vi "Save Config.vi"(8 "error in (no error)":errorcluster, 11 "MAS in":refnum<class "MAS.lvclass">) -> (0 "error out":errorcluster, 3 "MAS out":refnum<class "MAS.lvclass">)   [LabVIEW 2022 SP3, in "MAS.lvclass"]
uses:
  MAS.lvclass
  C:/Users/Josh.Thibeault/Desktop/MAS/Base/Base.lvclass
  Base/Base.lvclass/Base.ctl
  MAS.lvclass/MAS.ctl
  7da30ec2-8576-4118-b397-9a5033b99ef1.vi
  Base/Accessors/Read Config Path.vi
  Base/Accessors/Read Section.vi
  <vilib>/Utility/config.llb/Open Config Data.vi
  <userlib>/_OpenG.lib/variantconfig/variantconfig.llb/Write Section Cluster__ogtk.vi
  <vilib>/Utility/config.llb/Close Config Data.vi
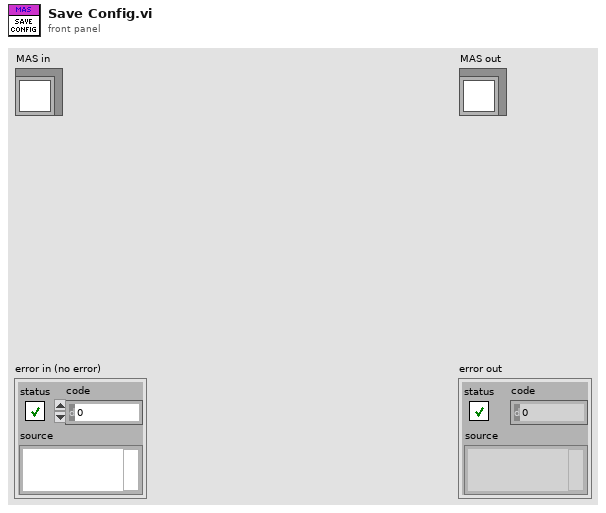
[diagram p1: front panel]
types:
  T1 = typedef "MAS.lvclass/Settings.ctl" = cluster{"Axis Name":string[]}
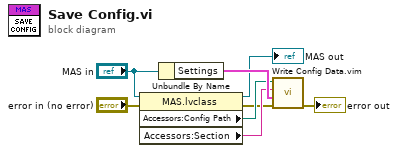
[diagram p0: block diagram]
diagram:
  n1 = property class="MAS.lvclass"(reference="MAS in", error in="error in (no error)") -> (reference out=→"MAS out":refnum<class "MAS.lvclass">, error out=w2:errorcluster, "Accessors:Config Path"=w5:path, "Accessors:Section"=w4:string)
  n2 = Unbundle By Name("MAS in") -> ("Settings"=w7:T1)
  n3 = call "Write Config Data.vim"("error in (no error)"=w2, "Section Formatted Cluster Type"=w7, "Section"=w4, "Config Path"=w5) -> ("error out"=→"error out":errorcluster)  [unwired: 7 in]
